vi "TEST_data_averaging.vi"() -> ()   [LabVIEW 2019]
panel:
  out "Boolean":bool
  out "Averaged Array":dbl[](array[numeric])
  out "Input":dbl[](array[numeric])
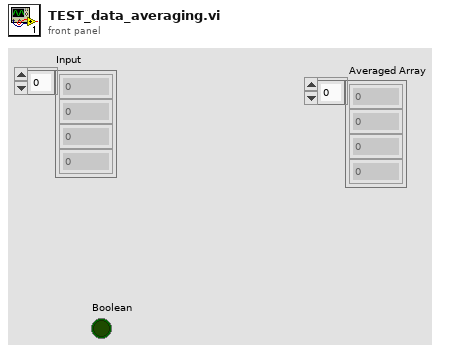
[diagram p1: front panel]
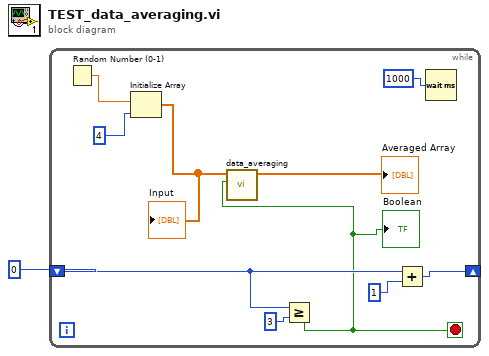
[diagram p0: block diagram]
diagram:
  n1 = while {
    shift-right: [w11] -> _
    shift-left: 0 -> [w9]
    stop <- w5 stop-if-true
    n2 = Random Number (0-1)() -> (number: 0 to 1=w4:dbl)
    n3 = Initialize Array(w4, 4) -> (w2:dbl[])
    "Input" <- w2
    n4 = Greater Or Equal?(x=w9, y=3) -> (x >= y?=w5:bool)
    "Boolean" <- w5
    n5 = call "data_averaging.vi"("Reset?"=w5, "New data"=w2) -> ("Output (averaged)"=→"Averaged Array":dbl[])  [unwired: 9 in]
    n6 = Add(x=w9, y=1) -> (x+y=w11:i32)
    n7 = Wait (ms)(milliseconds to wait=1000) -> ()  [unwired: 1 out]
  }
